vi "f_4_Tdon.vi"(0 "file path (IN)":path, 1 "Project #":string, 2 "Request #":string, 3 "TEST #":string, 5 "error in (no error)":errorcluster, 6 "VGE":dbl, 8 "ICE":dbl) -> (14 "file path (OUT)":path, 15 "Tdon (ns) (after filter)":dbl, 16 "DONE Tdon":bool, 19 "error out":errorcluster)   [LabVIEW 2020]
uses:
  GlobIndSw1.vi
  <vilib>/Waveform/WDTOps.llb/WDT Waveform Duration DBL.vi
  <vilib>/Waveform/WDTOps.llb/WDT Get Waveform Subset DBL.vi
  <vilib>/measure/mamon.llb/Trigger Detection for 1 Channel.vi
  <vilib>/measure/NI_MAPro.lvlib
  <vilib>/Analysis/NI_AALBase.lvlib
panel:
  in  "Decision ?":bool
  out "Cursor a : Channel 2 (after filter)":dbl
  out "Cursor a : Channel 1 (after filter)":dbl
  out "10% Vge (Theory)":dbl
  out "10% Ice (Theory)":dbl
  out "Waveform Graph":waveform(dbl)[](graph)
  out "Find Tdon":waveform(dbl)[](graph) caption="Tdon (ns)"
  # "Tdon = From 10% VGE to 10% ICE"
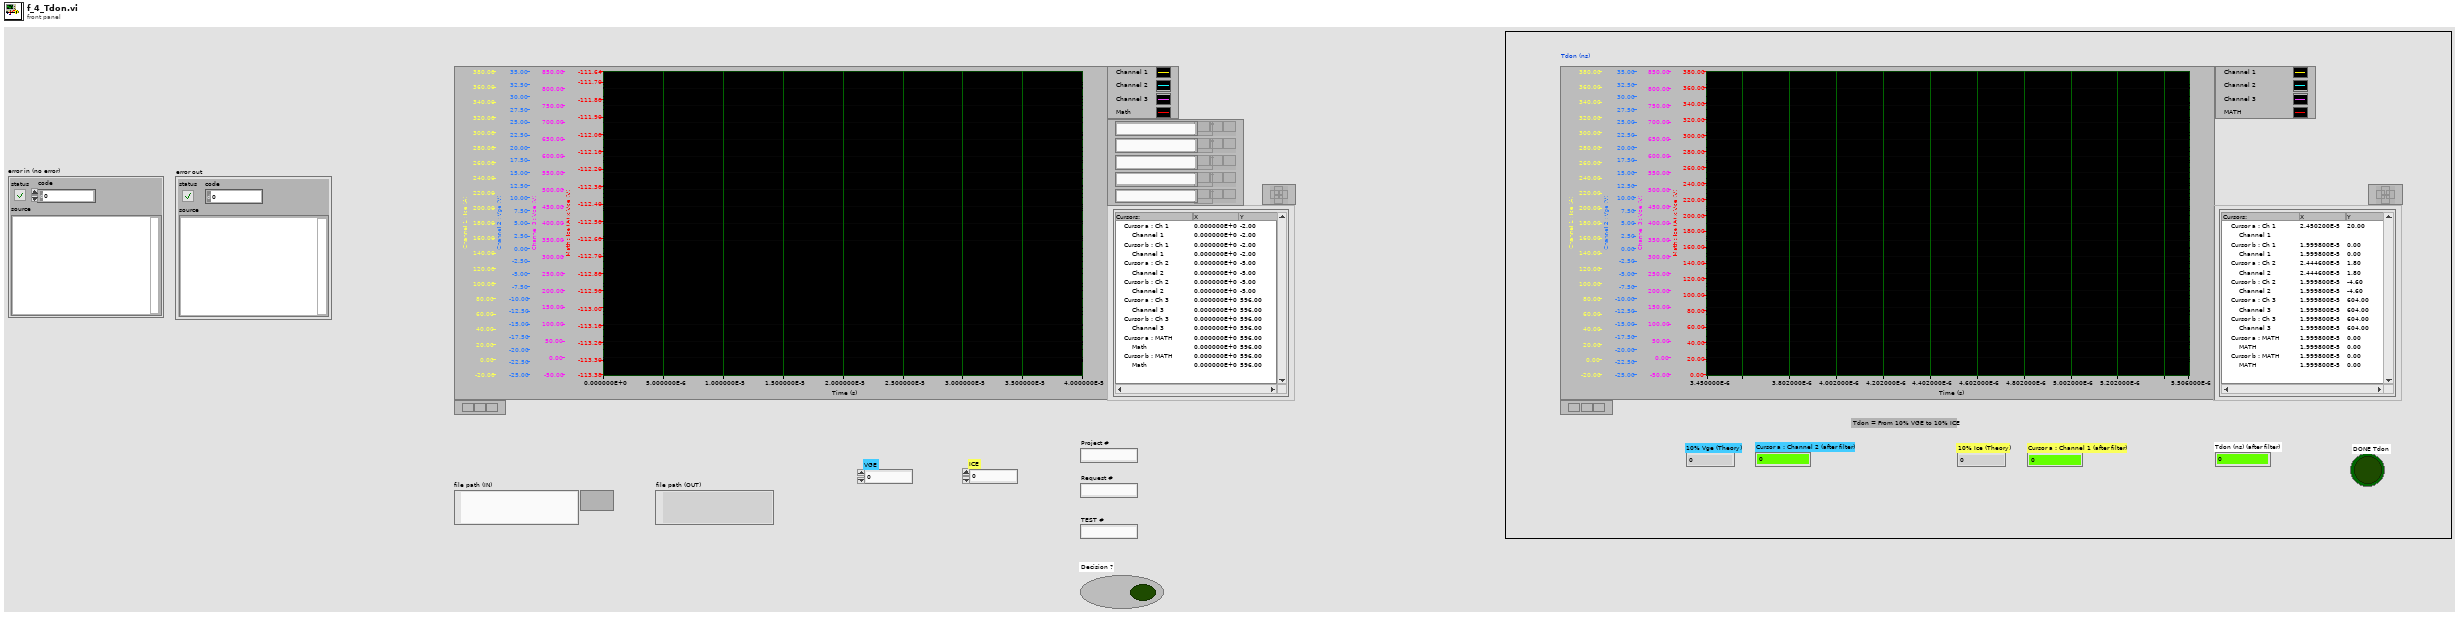
[diagram p1: front panel]
types:
  T1 = enum32{"Invalid", "Standard", "Closed", "Hidden", "Minimized", "Maximized"}
  T2 = typedef "imagedata.ctl" = cluster{"image type":i32, "image depth":i32, "image":u8[], "mask":u8[], "colors":u32[], "Rectangle":cluster{"left":i16, "top":i16, "right":i16, "bottom":i16}}
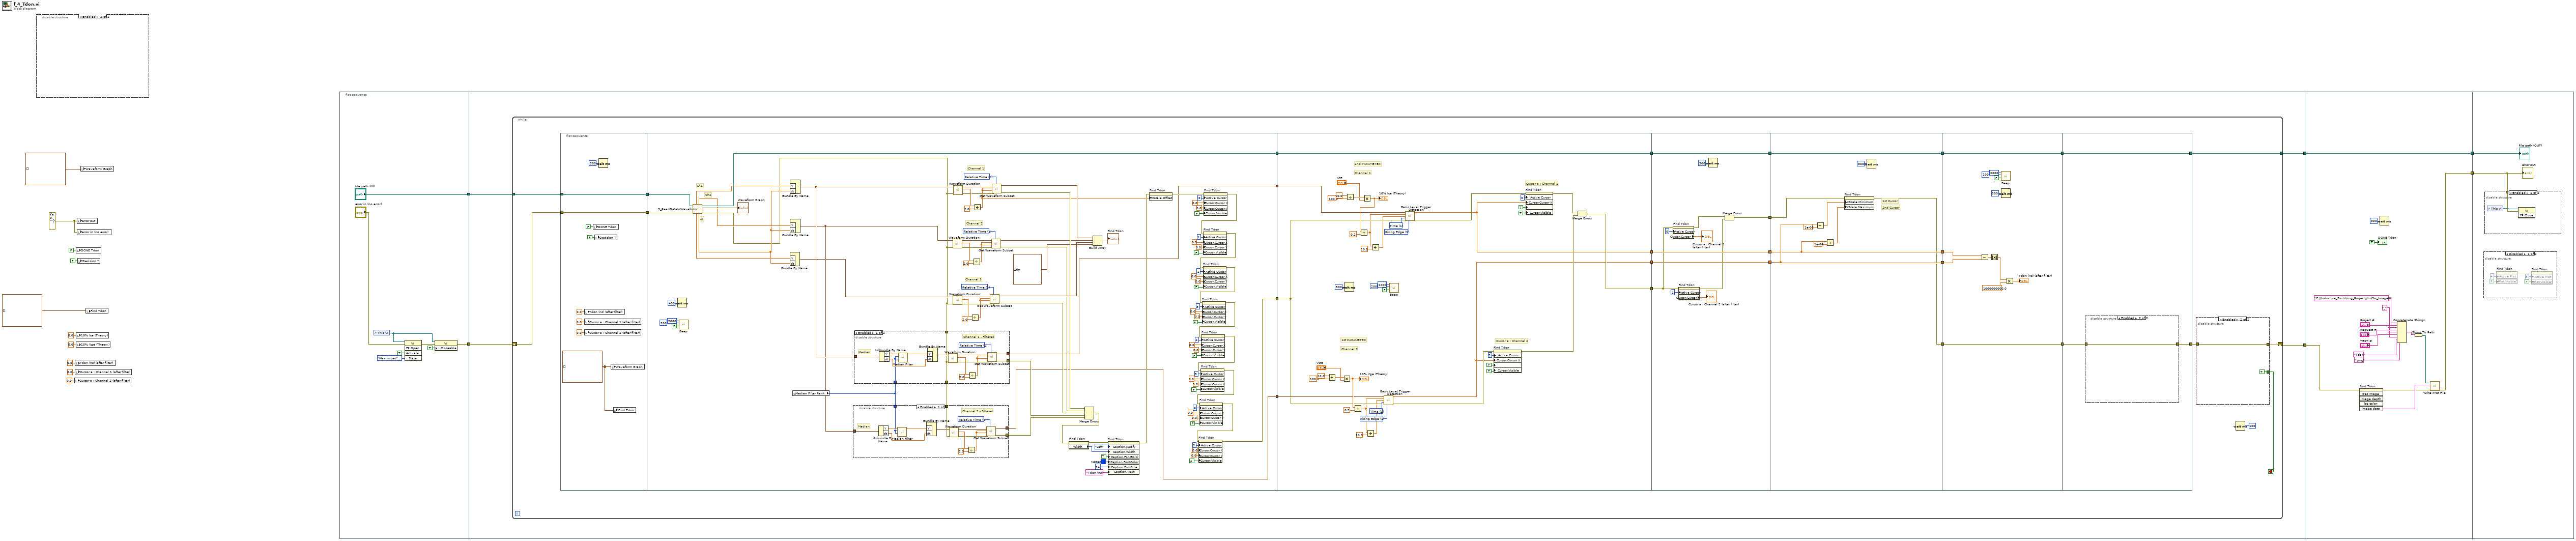
[diagram p0: block diagram]
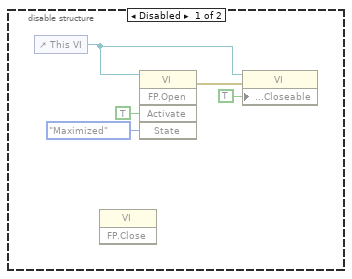
[diagram p2: hidden frame]
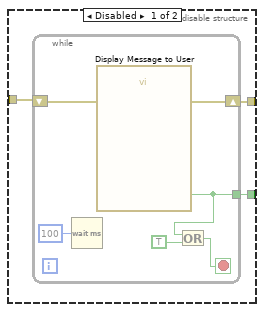
[diagram p3: hidden frame]
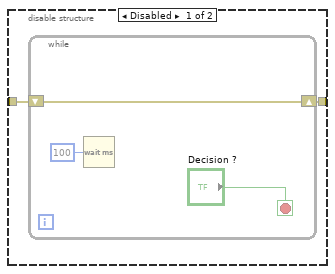
[diagram p6: hidden frame]
diagram:
  w9 = errorcluster {"status"=FALSE, "code"=0, "source"=""} ("error out")
  n1 = disable-structure shown="Enabled" {
    frame Disabled {
      n2 = control-ref of="This VI"() -> (w18:refnum<vi>)
      n3 = invoke class="VI" method="FP.Close"() -> (reference=w17:refnum<vi>)  [unwired: 2 in, 3 out]
      n4 = invoke class="VI" method="FP.Open"(reference=w18, "Activate"=TRUE ("Activate?"), "State"=T1."Maximized") -> (error in=w21:errorcluster, error out=w19:errorcluster)  [unwired: 1 in, 4 out]
      n5 = property class="VI"(reference=w18, error in=w19, "Front Panel.Closeable"=TRUE ("Front Panel Window:Closeable")) -> ()  [unwired: 2 out]
    }
    frame Enabled {
    }
  }
  n6 = local write "Cursor a : Channel 2 (after filter)"(0.0 ("Cursor a : Channel 2 (after filter)")) -> ()
  n7 = local write "Tdon (ns) (after filter)"(0.0 ("Tdon (ns) (after filter)")) -> ()
  n8 = local write "Cursor a : Channel 1 (after filter)"(0.0 ("Cursor a : Channel 1 (after filter)")) -> ()
  n9 = local write "DONE Tdon"(FALSE ("DONE Tdon")) -> ()
  n10 = local write "10% Ice (Theory)"(0.0 ("10% Ice (Theory)")) -> ()
  n11 = local write "10% Vge (Theory)"(0.0 ("10% Vge (Theory)")) -> ()
  n12 = local write "error out"(w9) -> ()
  n13 = local write "error in (no error)"(w9) -> ()
  n14 = local write "Decision ?"(FALSE ("Decision ?")) -> ()
  n15 = local write "Waveform Graph"(waveform(dbl)[] [] ("Waveform Graph")) -> ()
  n16 = local write "Find Tdon"(waveform(dbl)[] [] ("Tdon after Noise Filter")) -> ()
  n17 = flat-sequence {
    tunnel: ["file path (IN)"] -> w16
    tunnel: [w26] -> w15
    tunnel: [w34] -> w14
    tunnel: [w33] -> w13
    tunnel: w16 -> [w35]
    tunnel: w15 -> [w32]
    tunnel: w14 -> [w299]
    tunnel: [w302] -> w12
    tunnel: [w301] -> w11
    tunnel: w13 -> [w301]
    tunnel: w12 -> [w313]
    tunnel: w11 -> [w314]
    frame #0 {
      n18 = control-ref of="This VI"() -> (w30:refnum<vi>)
      n19 = invoke class="VI" method="FP.Open"(reference=w30, error in="error in (no error)", "Activate"=TRUE ("Activate?"), "State"=T1."Maximized") -> (error out=w31:errorcluster)  [unwired: 1 in, 4 out]
      n20 = property class="VI"(reference=w30, error in=w31, "Front Panel.Closeable"=TRUE ("Front Panel Window:Closeable")) -> (error out=w26:errorcluster)  [unwired: 1 out]
    }
    frame #1 {
      n21 = while {
        tunnel: w35 -> [w58]
        shift-right: [w40] -> w34
        shift-left: w32 -> [w57]
        tunnel: [w55] -> w33
        stop <- w39 stop-if-true
        n22 = flat-sequence {
          tunnel: [w81] -> w62
          tunnel: [w82] -> w61
          tunnel: w58 -> [w82]
          tunnel: w57 -> [w81]
          tunnel: w62 -> [w180]
          tunnel: w61 -> [w178]
          tunnel: [w174] -> w60
          tunnel: [w85] -> w51
          tunnel: [w84] -> w38
          tunnel: [w98] -> w37
          tunnel: w60 -> [w253]
          tunnel: [w253] -> w54
          tunnel: w51 -> [w235]
          tunnel: [w238] -> w50
          tunnel: [w233] -> w49
          tunnel: [w228] -> w48
          tunnel: w38 -> [w222]
          tunnel: w37 -> [w221]
          tunnel: w54 -> [w265]
          tunnel: [w265] -> w53
          tunnel: w50 -> [w254]
          tunnel: w49 -> [w262]
          tunnel: w48 -> [w261]
          tunnel: [w262] -> w47
          tunnel: [w261] -> w46
          tunnel: [w255] -> w45
          tunnel: w53 -> [w275]
          tunnel: [w275] -> w59
          tunnel: w47 -> [w268]
          tunnel: w46 -> [w271]
          tunnel: w45 -> [w266]
          tunnel: [w271] -> w44
          tunnel: [w268] -> w43
          tunnel: [w267] -> w41
          tunnel: w59 -> [w284]
          tunnel: [w284] -> w56
          tunnel: w44 -> [w278]
          tunnel: w43 -> [w279]
          tunnel: [w276] -> w42
          tunnel: w41 -> [w276]
          tunnel: [w288] -> w52
          tunnel: w56 -> [w290]
          tunnel: [w290] -> w55
          tunnel: w42 -> [w289]
          frame #0 {
            w77 = waveform(dbl)[] [] ("Waveform Graph")
            n23 = local write "Tdon (ns) (after filter)"(0.0 ("Tdon (ns) (after filter)")) -> ()
            n24 = local write "Cursor a : Channel 1 (after filter)"(0.0 ("Cursor a : Channel 1 (after filter)")) -> ()
            n25 = local write "Cursor a : Channel 2 (after filter)"(0.0 ("Cursor a : Channel 2 (after filter)")) -> ()
            n26 = local write "DONE Tdon"(FALSE ("DONE Tdon")) -> ()
            n27 = local write "Decision ?"(FALSE ("Decision ?")) -> ()
            n28 = Wait (ms)(milliseconds to wait=u32 300) -> ()  [unwired: 1 out]
            n29 = local write "Waveform Graph"(w77) -> ()
            n30 = local write "Find Tdon"(w77) -> ()
          }
          frame #1 {
            w172 = u16 1 items=["Samples", "Relative Time"] ("start/duration format")
            w161 = u16 1 items=["Samples", "Relative Time"] ("start/duration format")
            w160 = u16 1 items=["Samples", "Relative Time"] ("start/duration format")
            # "Channel 1"
            # "Channel 3"
            # "Channel 2"
            # "dt"
            # "Ch2"
            # "Ch1"
            n31 = Wait (ms)(milliseconds to wait=u32 400) -> ()  [unwired: 1 out]
            n32 = call <vilib>:"Beep.vi"("use system alert? (T)"=FALSE, "duration (msec)"=u32 200, "frequency (Hz)"=u32 2000) -> ()  [unwired: 9 in]
            n33 = call "3_ReadDatatoWaveform.vi"("error in (no error)"=w180, "file path (IN)"=w178) -> ("error out"=w90:errorcluster, "Waveform Graph"=→"Waveform Graph":waveform(dbl)[], "file path (OUT)"=w174:path, "dt"=w94:dbl, "Ch 2 Data"=w96:dbl[], "Ch 3 Data"=w95:dbl[], "Ch 1 Data"=w97:dbl[])  [unwired: 3 in]
            n34 = Bundle By Name("Y"=w95, "dt"=w94) -> (w93:waveform(dbl))  [unwired: 1 in]
            n35 = Bundle By Name("Y"=w97, "dt"=w94) -> (w92:waveform(dbl))  [unwired: 1 in]
            n36 = Bundle By Name("Y"=w96, "dt"=w94) -> (w91:waveform(dbl))  [unwired: 1 in]
            n37 = global read "GlobIndSw1.vi" "Median Filter Rank"() -> (w83:i32)
            n38 = disable-structure shown="Enabled" {
              disable-tunnel: w92 -> [w207 _]
              disable-tunnel: w90 -> [w199 _]
              disable-tunnel: [w199 _] -> w89
              disable-tunnel: [w198 _] -> w88
              disable-tunnel: [w197 _] -> w85
              disable-tunnel: w83 -> [w196 _]
              frame Enabled {
                w201 = u16 1 items=["Samples", "Relative Time"] ("start/duration format")
                # "Channel 1 - Filtered"
                # "Median"
                n39 = Unbundle By Name(w207) -> ("Y"=w210:dbl[], "dt"=w208:dbl)
                n40 = call <vilib>:"Median Filter.vi"("right rank"=w196, "left rank"=w196, "X"=w210) -> ("Filtered X"=w209:dbl[])  [unwired: 7 in, 1 out]
                n41 = Bundle By Name("Y"=w209, "dt"=w208) -> (w200:waveform(dbl))  [unwired: 1 in]
                n42 = call-poly <vilib>:"Waveform Duration.vi"("error in (no error)"=w199, "waveform in"=w200) -> ("error out"=w204:errorcluster, "duration"=w206:dbl, "waveform out"=w205:waveform(dbl))  [unwired: 7 in]
                n43 = Divide(x=w206, y=2.0) -> (x/y=w203:dbl)
                n44 = call-poly <vilib>:"Get Waveform Subset.vi"("start/duration format"=w201, "error in (no error)"=w204, "duration"=w203, "start samples/time"=w203, "waveform in"=w205) -> ("error out"=w198:errorcluster, "waveform out"=w197:waveform(dbl))  [unwired: 1 in, 2 out]
              }
              frame Disabled {
              }
            }
            n45 = disable-structure shown="Enabled" {
              disable-tunnel: w91 -> [w192 _]
              disable-tunnel: w89 -> [w184 _]
              disable-tunnel: [w183 _] -> w87
              disable-tunnel: [w182 _] -> w84
              disable-tunnel: w83 -> [w181 _]
              frame Enabled {
                w186 = u16 1 items=["Samples", "Relative Time"] ("start/duration format")
                # "Channel 2 - Filtered"
                # "Median"
                n46 = Unbundle By Name(w192) -> ("Y"=w195:dbl[], "dt"=w193:dbl)
                n47 = call <vilib>:"Median Filter.vi"("right rank"=w181, "left rank"=w181, "X"=w195) -> ("Filtered X"=w194:dbl[])  [unwired: 7 in, 1 out]
                n48 = Bundle By Name("Y"=w194, "dt"=w193) -> (w185:waveform(dbl))  [unwired: 1 in]
                n49 = call-poly <vilib>:"Waveform Duration.vi"("error in (no error)"=w184, "waveform in"=w185) -> ("error out"=w189:errorcluster, "duration"=w191:dbl, "waveform out"=w190:waveform(dbl))  [unwired: 7 in]
                n50 = Divide(x=w191, y=2.0) -> (x/y=w188:dbl)
                n51 = call-poly <vilib>:"Get Waveform Subset.vi"("start/duration format"=w186, "error in (no error)"=w189, "duration"=w188, "start samples/time"=w188, "waveform in"=w190) -> ("error out"=w183:errorcluster, "waveform out"=w182:waveform(dbl))  [unwired: 1 in, 2 out]
              }
              frame Disabled {
              }
            }
            n52 = call-poly <vilib>:"Waveform Duration.vi"("error in (no error)"=w90, "waveform in"=w91) -> ("error out"=w166:errorcluster, "duration"=w163:dbl, "waveform out"=w165:waveform(dbl))  [unwired: 7 in]
            n53 = call-poly <vilib>:"Waveform Duration.vi"("error in (no error)"=w90, "waveform in"=w93) -> ("error out"=w167:errorcluster, "duration"=w170:dbl, "waveform out"=w168:waveform(dbl))  [unwired: 7 in]
            n54 = call-poly <vilib>:"Waveform Duration.vi"("error in (no error)"=w90, "waveform in"=w92) -> ("error out"=w156:errorcluster, "duration"=w159:dbl, "waveform out"=w157:waveform(dbl))  [unwired: 7 in]
            n55 = Divide(x=w170, y=2.0) -> (x/y=w171:dbl)
            n56 = Divide(x=w163, y=2.0) -> (x/y=w162:dbl)
            n57 = Divide(x=w159, y=2.0) -> (x/y=w141:dbl)
            n58 = call-poly <vilib>:"Get Waveform Subset.vi"("start/duration format"=w172, "error in (no error)"=w167, "duration"=w171, "start samples/time"=w171, "waveform in"=w168) -> ("error out"=w150:errorcluster, "waveform out"=w153:waveform(dbl))  [unwired: 1 in, 2 out]
            n59 = call-poly <vilib>:"Get Waveform Subset.vi"("start/duration format"=w161, "error in (no error)"=w166, "duration"=w162, "start samples/time"=w162, "waveform in"=w165) -> ("error out"=w151:errorcluster, "waveform out"=w99:waveform(dbl))  [unwired: 1 in, 2 out]
            n60 = call-poly <vilib>:"Get Waveform Subset.vi"("start/duration format"=w160, "error in (no error)"=w156, "duration"=w141, "start samples/time"=w141, "waveform in"=w157) -> ("error out"=w152:errorcluster, "waveform out"=w154:waveform(dbl))  [unwired: 1 in, 2 out]
            n61 = Merge Errors(w152, w151, w150, w88, w87) -> (w149:errorcluster)
            n62 = property on="Find Tdon" class="WFGraph (strict)"(error in=w149) -> (error out=w143:errorcluster, "Width"=w142:u32)  [unwired: 1 in, 1 out]
            n63 = Build Array(w154, w99, w153, waveform(dbl) {"t0"=timestamp(0 s since 1904-01-01), "dt"=1.0, "Y"=[]} ("element")) -> (→"Find Tdon":waveform(dbl)[])
            n64 = property on="Find Tdon" class="WFGraph (strict)"(error in=w143, "Caption.Justify"=enum16{"Left", "Center", "Right"}."Left" ("Caption.Justification"), "Caption.Width"=w142, "Caption.FontBold"=TRUE ("Caption.Font:Bold"), "Caption.FontColor"=u32 16860 ("Caption.Font:Color"), "Caption.FontSize"=u32 24 ("Caption.Font:Size"), "Caption.Text"="Tdon (ns)") -> (error out=w140:errorcluster)  [unwired: 1 in, 1 out]
            n65 = property on="Find Tdon" class="WFGraph (strict)"(error in=w140, "XScale.Offset"=w141) -> (error out=w107:errorcluster)  [unwired: 1 in, 1 out]
            n66 = property on="Find Tdon" class="WFGraph (strict)"(error in=w107, "Active Cursor"=u32 0, "Cursor.Cursor X"=0.0 ("Cursor.Cursor Position:Cursor X"), "Cursor.Cursor Y"=0.0 ("Cursor.Cursor Position:Cursor Y"), "Cursor.Visible"=FALSE) -> (error out=w106:errorcluster)  [unwired: 1 in, 1 out]
            n67 = property on="Find Tdon" class="WFGraph (strict)"(error in=w106, "Active Cursor"=u32 1, "Cursor.Cursor X"=0.0 ("Cursor.Cursor Position:Cursor X"), "Cursor.Cursor Y"=0.0 ("Cursor.Cursor Position:Cursor Y"), "Cursor.Visible"=FALSE) -> (error out=w105:errorcluster)  [unwired: 1 in, 1 out]
            n68 = property on="Find Tdon" class="WFGraph (strict)"(error in=w105, "Active Cursor"=u32 2, "Cursor.Cursor X"=0.0 ("Cursor.Cursor Position:Cursor X"), "Cursor.Cursor Y"=0.0 ("Cursor.Cursor Position:Cursor Y"), "Cursor.Visible"=FALSE) -> (error out=w104:errorcluster)  [unwired: 1 in, 1 out]
            n69 = property on="Find Tdon" class="WFGraph (strict)"(error in=w104, "Active Cursor"=u32 3, "Cursor.Cursor X"=0.0 ("Cursor.Cursor Position:Cursor X"), "Cursor.Cursor Y"=0.0 ("Cursor.Cursor Position:Cursor Y"), "Cursor.Visible"=FALSE) -> (error out=w103:errorcluster)  [unwired: 1 in, 1 out]
            n70 = property on="Find Tdon" class="WFGraph (strict)"(error in=w103, "Active Cursor"=u32 4, "Cursor.Cursor X"=0.0 ("Cursor.Cursor Position:Cursor X"), "Cursor.Cursor Y"=0.0 ("Cursor.Cursor Position:Cursor Y"), "Cursor.Visible"=FALSE) -> (error out=w102:errorcluster)  [unwired: 1 in, 1 out]
            n71 = property on="Find Tdon" class="WFGraph (strict)"(error in=w102, "Active Cursor"=u32 5, "Cursor.Cursor X"=0.0 ("Cursor.Cursor Position:Cursor X"), "Cursor.Cursor Y"=0.0 ("Cursor.Cursor Position:Cursor Y"), "Cursor.Visible"=FALSE) -> (error out=w101:errorcluster)  [unwired: 1 in, 1 out]
            n72 = property on="Find Tdon" class="WFGraph (strict)"(error in=w101, "Active Cursor"=u32 6, "Cursor.Cursor X"=0.0 ("Cursor.Cursor Position:Cursor X"), "Cursor.Cursor Y"=0.0 ("Cursor.Cursor Position:Cursor Y"), "Cursor.Visible"=FALSE) -> (error out=w100:errorcluster)  [unwired: 1 in, 1 out]
            n73 = property on="Find Tdon" class="WFGraph (strict)"(error in=w100, "Active Cursor"=u32 7, "Cursor.Cursor X"=0.0 ("Cursor.Cursor Position:Cursor X"), "Cursor.Cursor Y"=0.0 ("Cursor.Cursor Position:Cursor Y"), "Cursor.Visible"=FALSE) -> (error out=w98:errorcluster)  [unwired: 1 in, 1 out]
          }
          frame #2 {
            w226 = u16 1 items=["Falling Edge", "Rising Edge"] ("trigger slope")
            w227 = u16 1 items=["Index", "Time"] ("location mode")
            w236 = u16 1 items=["Falling Edge", "Rising Edge"] ("trigger slope")
            w237 = u16 1 items=["Index", "Time"] ("location mode")
            # "Cursor a : Channel 1"
            # "2nd PARAMETER"
            # "Channel 1"
            # "Cursor a : Channel 2"
            # "1st PARAMETER"
            # "Channel 2"
            n74 = Divide(x=10.0, y=100.0) -> (x/y=w251:dbl)
            n75 = Multiply(x=w251, y="VGE") -> (x*y=w230:dbl)
            "10% Vge (Theory)" <- w230
            n76 = Wait (ms)(milliseconds to wait=u32 500) -> ()  [unwired: 1 out]
            n77 = Divide(x=10.0, y=100.0) -> (x/y=w244:dbl)
            n78 = Add(x=w230, y=0.2) -> (x+y=w216:dbl)
            n79 = Multiply(x=w244, y="ICE") -> (x*y=w231:dbl)
            "10% Ice (Theory)" <- w231
            n80 = Add(x=w231, y=0.2) -> (x+y=w219:dbl)
            n81 = Divide(x=w216, y=10.0) -> (x/y=w215:dbl)
            n82 = Divide(x=w219, y=10.0) -> (x/y=w218:dbl)
            n83 = call-poly <vilib>:"Basic Level Trigger Detection.vi"("signal in"=w222, "level"=w216, "hysteresis"=w215, "location mode"=w227, "error in (no error)"=w221, "trigger slope"=w226) -> ("trigger location"=w228:dbl, "error out"=w229:errorcluster)  [unwired: 7 in, 1 out]
            n84 = call <vilib>:"Beep.vi"("use system alert? (T)"=FALSE, "duration (msec)"=u32 200, "frequency (Hz)"=u32 2000) -> ()  [unwired: 9 in]
            n85 = call-poly <vilib>:"Basic Level Trigger Detection.vi"("signal in"=w235, "level"=w219, "hysteresis"=w218, "location mode"=w237, "error in (no error)"=w221, "trigger slope"=w236) -> ("trigger location"=w233:dbl, "error out"=w234:errorcluster)  [unwired: 7 in, 1 out]
            n86 = property on="Find Tdon" class="WFGraph (strict)"(error in=w229, "Active Cursor"=u32 2, "Cursor.Cursor X"=w228, "Cursor.Cursor Name Visible"=TRUE, "Cursor.Visible"=TRUE) -> (error out=w240:errorcluster)  [unwired: 1 in, 1 out]
            n87 = property on="Find Tdon" class="WFGraph (strict)"(error in=w234, "Active Cursor"=u32 0, "Cursor.Cursor X"=w233, "Cursor.Cursor Name Visible"=TRUE, "Cursor.Visible"=TRUE) -> (error out=w239:errorcluster)  [unwired: 1 in, 1 out]
            n88 = Merge Errors(w239, w240) -> (w238:errorcluster)
          }
          frame #3 {
            n89 = property on="Find Tdon" class="WFGraph (strict)"(error in=w254, "Active Cursor"=u32 0) -> (error out=w260:errorcluster, "Cursor.Cursor Y"=→"Cursor a : Channel 1 (after filter)":dbl)  [unwired: 1 in, 1 out]
            n90 = property on="Find Tdon" class="WFGraph (strict)"(error in=w254, "Active Cursor"=u32 2) -> (error out=w259:errorcluster, "Cursor.Cursor Y"=→"Cursor a : Channel 2 (after filter)":dbl)  [unwired: 1 in, 1 out]
            n91 = Wait (ms)(milliseconds to wait=u32 300) -> ()  [unwired: 1 out]
            n92 = Merge Errors(w260, w259) -> (w255:errorcluster)
          }
          frame #4 {
            # "2nd Cursor"
            # "1st Cursor"
            n93 = Subtract(x=w271, y=1e-06) -> (x-y=w270:dbl)
            n94 = Add(x=w268, y=1e-06) -> (x+y=w269:dbl)
            n95 = property on="Find Tdon" class="WFGraph (strict)"(error in=w266, "XScale.Minimum"=w270, "XScale.Maximum"=w269) -> (error out=w267:errorcluster)  [unwired: 1 in, 1 out]
            n96 = Wait (ms)(milliseconds to wait=u32 300) -> ()  [unwired: 1 out]
          }
          frame #5 {
            n97 = Subtract(x=w279, y=w278) -> (x-y=w281:dbl)
            n98 = Absolute Value(x=w281) -> (abs(x)=w282:dbl)
            n99 = call <vilib>:"Beep.vi"("use system alert? (T)"=FALSE, "duration (msec)"=u32 200, "frequency (Hz)"=u32 2000) -> ()  [unwired: 9 in]
            n100 = Wait (ms)(milliseconds to wait=u32 300) -> ()  [unwired: 1 out]
            n101 = Multiply(x=w282, y=1000000000.0) -> (x*y=→"Tdon (ns) (after filter)":dbl)
          }
          frame #6 {
            n102 = disable-structure shown="Enabled" {
              disable-tunnel: w289 -> [w292 w296]
              disable-tunnel: [w291 w296] -> w288
              frame Disabled {
                n103 = while {
                  shift-right: [w293] -> w291
                  shift-left: w292 -> [w293]
                  stop <- "Decision ?" stop-if-true
                  n104 = Wait (ms)(milliseconds to wait=u32 100) -> ()  [unwired: 1 out]
                }
              }
              frame Enabled {
              }
            }
          }
        }
        n105 = disable-structure shown="Enabled" {
          disable-tunnel: w52 -> [w65 w73]
          disable-tunnel: [w64 w73] -> w40
          disable-tunnel: [w63 TRUE ("NO")] -> w39
          frame Disabled {
            n106 = while {
              tunnel: [w67] -> w63
              shift-right: [w70] -> w64
              shift-left: w65 -> [w71]
              stop <- w69 stop-if-true
              n107 = Wait (ms)(milliseconds to wait=u32 100) -> ()  [unwired: 1 out]
              n108 = call "Display Message to User"("error in (no error)"=w71) -> ("error out"=w70:errorcluster, "NO"=w67:bool)  [unwired: 9 in]
              n109 = Or(x=w67, y=TRUE) -> (x .or. y?=w69:bool)
            }
          }
          frame Enabled {
          }
        }
        n110 = Wait (ms)(milliseconds to wait=u32 100) -> ()  [unwired: 1 out]
      }
    }
    frame #2 {
      w305 = "_"
      n111 = invoke on="Find Tdon" class="WFGraph (strict)" method="Get Image"(error in=w299) -> (error out=w298:errorcluster, "image data"=w300:T2)  [unwired: 5 in, 4 out]
      n112 = Wait (ms)(milliseconds to wait=u32 300) -> ()  [unwired: 1 out]
      n113 = Concatenate Strings("C:\\Inductive_Switching_Project\\IndSw_Image\\" ("string"), "Project #", w305, "Request #", w305, "TEST #", w305, "Tdon" ("string"), ".png" ("string")) -> (w310:string)
      n114 = String To Path(string=w310) -> (path=w309:path)
      n115 = call <vilib>:"Write PNG File.vi"("error in (no error)"=w298, "image data"=w300, "path to PNG file"=w309) -> ("error out"=w302:errorcluster)  [unwired: 7 in, 1 out]
      "DONE Tdon" <- TRUE ("DONE Tdon")
    }
    frame #3 {
      n116 = disable-structure shown="Disabled" {
        frame Disabled {
          n117 = property on="Find Tdon" class="WFGraph (strict)"("Active Plot"=u32 4, "Plot.Visible?"=FALSE ("Plot.Visible")) -> (error out=w315:errorcluster)  [unwired: 2 in, 1 out]
          n118 = property on="Find Tdon" class="WFGraph (strict)"(error in=w315, "Active Plot"=u32 5, "Plot.Visible?"=FALSE ("Plot.Visible")) -> ()  [unwired: 1 in, 2 out]
        }
        frame Enabled {
        }
      }
      n119 = disable-structure shown="Enabled" {
        disable-tunnel: w313 -> [w320 _]
        frame Enabled {
          n120 = control-ref of="This VI"() -> (w321:refnum<vi>)
          n121 = invoke class="VI" method="FP.Close"(reference=w321, error in=w320) -> ()  [unwired: 1 in, 3 out]
        }
        frame Disabled {
        }
      }
      "error out" <- w313
      "file path (OUT)" <- w314
    }
  }
